vi "UpdateTask.vi"(8 "error in (no error)":errorcluster, 9 "Params":T1={"Mice ID"=[], "ExpType"=[], "Trial Interval"=[], "Pulse Duration"=[158.0, 152.0, 156.0, 167.0, 172.0], "microL_per_pulse"=[6.0, 6.0, 6.0, 6.0, 6.0], "Response Interval"=[1000.0, 1000.0, 1000.0, 1000.0, 1000.0], "Bad Delay"=[], "Response Period"=[], "liquid_type"="water", "Stimuli"=[], "Rewarded Stimuli"=[], "AirDur"=[]} {"AirDur" format="%#_13g"}, 10 "Task":dbl[](array[numeric]), 11 "Acquisition in":refnum<class "Acquisition.lvclass">) -> (0 "error out":errorcluster, 1 "Change":bool, 2 "Params 2":T1={"Mice ID"=[], "ExpType"=[], "Trial Interval"=[], "Pulse Duration"=[158.0, 152.0, 156.0, 167.0, 172.0], "microL_per_pulse"=[6.0, 6.0, 6.0, 6.0, 6.0], "Response Interval"=[1000.0, 1000.0, 1000.0, 1000.0, 1000.0], "Bad Delay"=[], "Response Period"=[], "liquid_type"="water", "Stimuli"=[], "Rewarded Stimuli"=[], "AirDur"=[]} {"AirDur" format="%#_13g"}, 3 "Acquisition out":refnum<class "Acquisition.lvclass">)   [LabVIEW 2014, in "Acquisition.lvclass"]
uses:
  Acquisition.lvclass
  ParamsArray.ctl
  Acquisition.lvclass/Acquisition.ctl
  Database/Database.lvclass
panel:
  out "task params":T2(array[cluster])
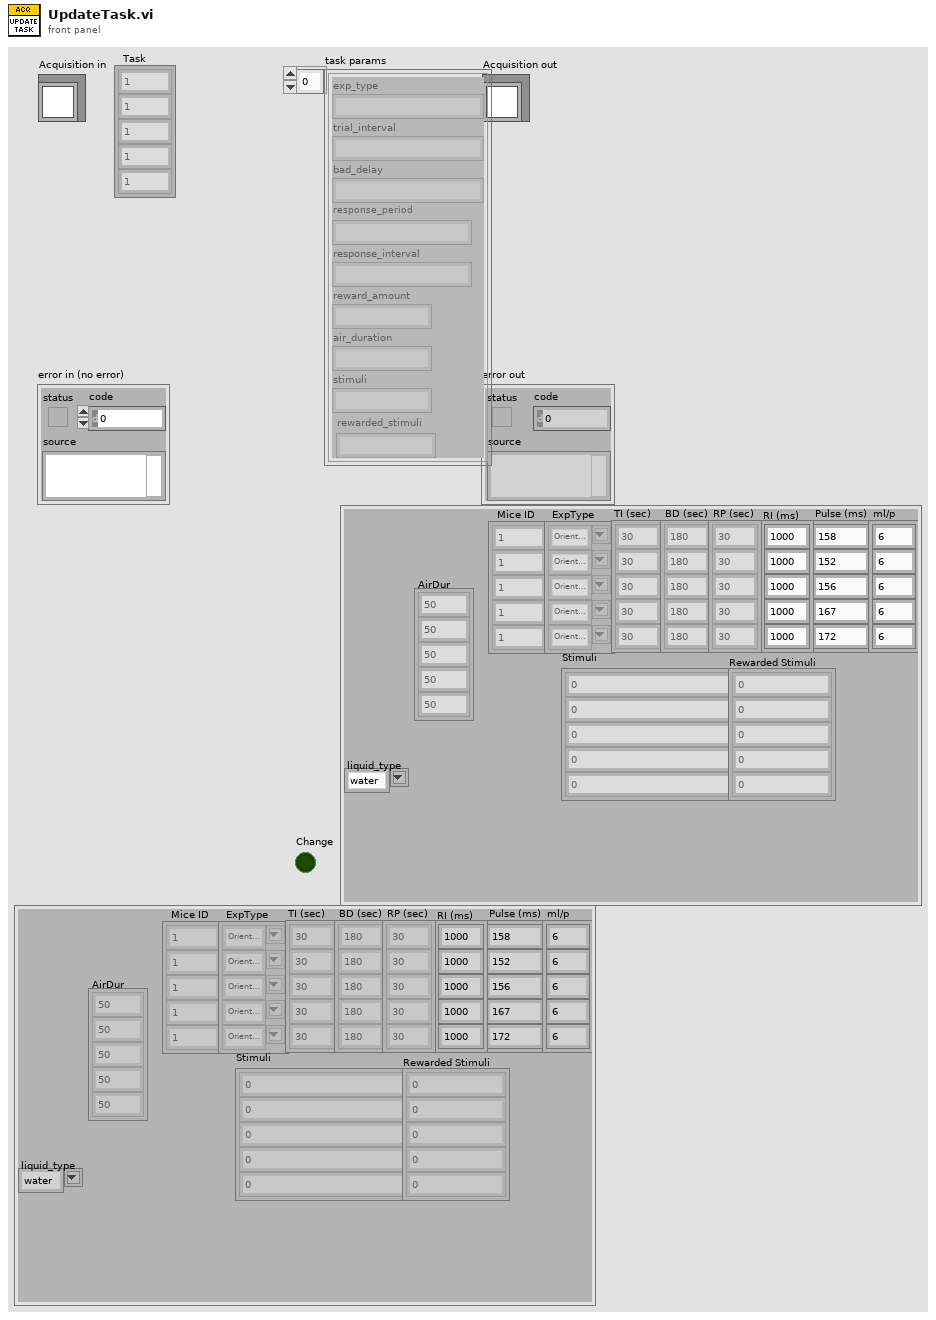
[diagram p1: front panel]
types:
  T1 = typedef "ParamsArray.ctl" = cluster{"Mice ID":dbl[], "ExpType":string[], "Trial Interval":dbl[], "Pulse Duration":dbl[], "microL_per_pulse":dbl[], "Response Interval":dbl[], "Bad Delay":dbl[], "Response Period":dbl[], "liquid_type":string, "Stimuli":string[], "Rewarded Stimuli":string[], "AirDur":dbl[]}
  T2 = cluster{"exp_type":string, "trial_interval":string, "bad_delay":string, "response_period":string, "response_interval":string, "reward_amount":string, "air_duration":string, "stimuli":string, "rewarded_stimuli":string}[]
  T3 = cluster{"exp_type":string, "trial_interval":string, "bad_delay":string, "response_period":string, "response_interval":string, "reward_amount":string, "air_duration":string, "stimuli":string, "rewarded_stimuli":string}
  T4 = cluster{"Mice ID":bool[], "ExpType":bool[], "Trial Interval":bool[], "Pulse Duration":bool[], "microL_per_pulse":bool[], "Response Interval":bool[], "Bad Delay":bool[], "Response Period":bool[], "liquid_type":bool, "Stimuli":bool[], "Rewarded Stimuli":bool[], "AirDur":bool[]}
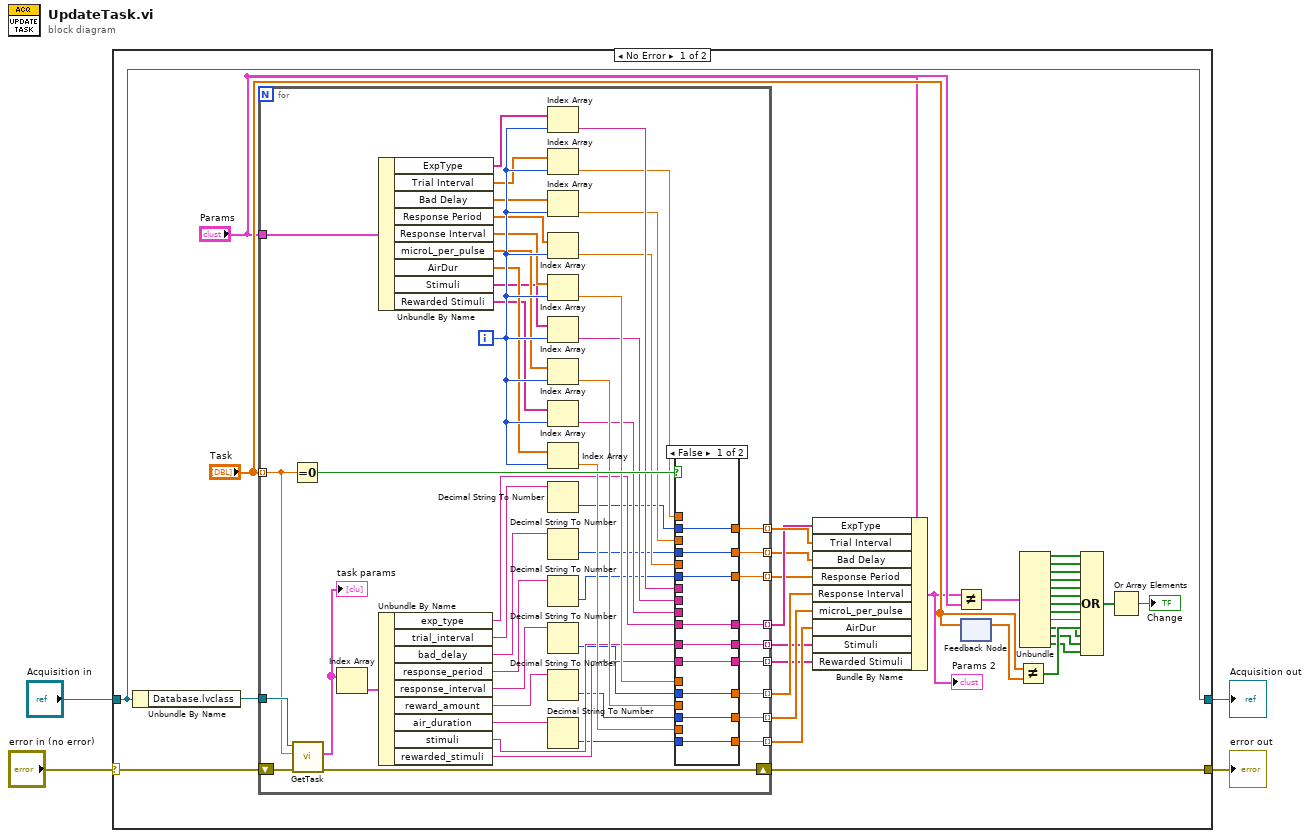
[diagram p0: block diagram]
diagram:
  n1 = case shown="No Error" "error in (no error)" {
    selector: "error in (no error)" -> [w35 w108]
    tunnel: [w37 w107] -> w2
    tunnel: "Acquisition in" -> [w37 w107]
    tunnel: [w34 w108] -> w1
    frame No Error {
      n2 = Unbundle By Name(w37) -> ("Database.lvclass"=w36:refnum<class "Database.lvclass">)
      n3 = for {
        tunnel: w36 -> [w88]
        shift-right: [w86] -> w34
        shift-left: w35 -> [w87]
        tunnel: "Task" -> [w61] mode=indexing
        tunnel: "Params" -> [w83]
        tunnel: [w40] -> w32 mode=indexing
        tunnel: [w46] -> w33 mode=indexing
        tunnel: [w45] -> w31 mode=indexing
        tunnel: [w44] -> w30 mode=indexing
        tunnel: [w43] -> w28 mode=indexing
        tunnel: [w42] -> w27 mode=indexing
        tunnel: [w41] -> w29 mode=indexing
        tunnel: [w39] -> w26 mode=indexing
        tunnel: [w38] -> w23 mode=indexing
        i -> [w81]
        n4 = Equal To 0?(x=w61) -> (x = 0?=w82:bool)
        n5 = call-dynamic "GetTask.vi"("error in (no error)"=w87, "task"=w61, "Database in"=w88) -> ("error out"=w86:errorcluster, "task params"=w85:T2)  [unwired: 6 in, 1 out]
        "task params" <- w85
        n6 = Index Array(array=w85) -> (element=w84:T3)  [unwired: 1 in]
        n7 = Unbundle By Name(w83) -> ("ExpType"=w80:string[], "Trial Interval"=w79:dbl[], "Bad Delay"=w78:dbl[], "Response Period"=w77:dbl[], "Response Interval"=w76:dbl[], "microL_per_pulse"=w75:dbl[], "AirDur"=w74:dbl[], "Stimuli"=w73:string[], "Rewarded Stimuli"=w72:string[])
        n8 = Unbundle By Name(w84) -> ("exp_type"=w62:string, "trial_interval"=w58:string, "bad_delay"=w56:string, "response_period"=w54:string, "response_interval"=w52:string, "reward_amount"=w50:string, "air_duration"=w48:string, "stimuli"=w60:string, "rewarded_stimuli"=w59:string)
        n9 = Index Array(array=w80, index=w81) -> (element=w71:string)
        n10 = Index Array(array=w79, index=w81) -> (element=w70:dbl)
        n11 = Index Array(array=w78, index=w81) -> (element=w69:dbl)
        n12 = Index Array(array=w77, index=w81) -> (element=w68:dbl)
        n13 = Index Array(array=w76, index=w81) -> (element=w67:dbl)
        n14 = Index Array(array=w73, index=w81) -> (element=w64:string)
        n15 = Index Array(array=w75, index=w81) -> (element=w66:dbl)
        n16 = Index Array(array=w72, index=w81) -> (element=w63:string)
        n17 = Index Array(array=w74, index=w81) -> (element=w65:dbl)
        n18 = Decimal String To Number(string=w58) -> (number=w57:i32)  [unwired: 2 in, 1 out]
        n19 = Decimal String To Number(string=w56) -> (number=w55:i32)  [unwired: 2 in, 1 out]
        n20 = Decimal String To Number(string=w54) -> (number=w53:i32)  [unwired: 2 in, 1 out]
        n21 = Decimal String To Number(string=w52) -> (number=w51:i32)  [unwired: 2 in, 1 out]
        n22 = Decimal String To Number(string=w50) -> (number=w49:i32)  [unwired: 2 in, 1 out]
        n23 = Decimal String To Number(string=w48) -> (number=w47:i32)  [unwired: 2 in, 1 out]
        n24 = case shown="False" w82 {
          tunnel: w71 -> [_ w106]
          tunnel: w70 -> [_ w105]
          tunnel: w69 -> [_ w104]
          tunnel: w68 -> [_ w103]
          tunnel: w67 -> [_ w102]
          tunnel: w66 -> [_ w101]
          tunnel: w65 -> [_ w100]
          tunnel: w64 -> [_ w99]
          tunnel: w63 -> [_ w98]
          tunnel: [w97 w106] -> w40
          tunnel: [w94 w105] -> w46
          tunnel: [w93 w104] -> w45
          tunnel: [w92 w103] -> w44
          tunnel: [w91 w102] -> w43
          tunnel: [w90 w101] -> w42
          tunnel: [w89 w100] -> w41
          tunnel: [w96 w99] -> w39
          tunnel: [w95 w98] -> w38
          tunnel: w62 -> [w97 _]
          tunnel: w60 -> [w96 _]
          tunnel: w59 -> [w95 _]
          tunnel: w57 -> [w94 _]
          tunnel: w55 -> [w93 _]
          tunnel: w53 -> [w92 _]
          tunnel: w51 -> [w91 _]
          tunnel: w49 -> [w90 _]
          tunnel: w47 -> [w89 _]
          frame False {
          }
          frame True {
          }
        }
      }
      n25 = Bundle By Name(cluster="Params", "ExpType"=w32, "Trial Interval"=w33, "Bad Delay"=w31, "Response Period"=w30, "Response Interval"=w28, "microL_per_pulse"=w27, "AirDur"=w29, "Stimuli"=w26, "Rewarded Stimuli"=w23) -> (w5:T1)
      "Params 2" <- w5
      n26 = Not Equal?(x=w5, y="Params") -> (x != y?=w18:T4)
      n27 = feedback #1() -> (w21:dbl[])  [unwired: 1 in]
      n28 = feedback-in #1("Task") -> ()
      n29 = Not Equal?(x="Task", y=w21) -> (x != y?=w22:bool[])
      n30 = Unbundle(w18) -> ("Mice ID"=w17:bool[], "ExpType"=w16:bool[], "Trial Interval"=w15:bool[], "Pulse Duration"=w14:bool[], "microL_per_pulse"=w13:bool[], "Response Interval"=w12:bool[], "Bad Delay"=w11:bool[], "Response Period"=w10:bool[], "liquid_type"=w9:bool, "Stimuli"=w8:bool[], "Rewarded Stimuli"=w7:bool[], "AirDur"=w6:bool[])
      n31 = Compound Arithmetic op=OR(w17, w16, w15, w14, w13, w12, w11, w10, w9, w22, w8, w7, w6) -> (w25:bool[])
      n32 = Or Array Elements(Boolean array=w25) -> (logical OR=→"Change":bool)
    }
    frame Error {
    }
  }
  "error out" <- w1
  "Acquisition out" <- w2
